vi "Set Options.vi"(8 "error in":errorcluster, 10 "WebSocket reference":refnum<class "WebSocket Client.lvclass">, 11 "Websocket Handler in":refnum<class "Websocket Handler.lvclass">) -> (0 "error out":errorcluster, 2 "reference out":refnum<class "WebSocket Client.lvclass">, 3 "Websocket Handler out":refnum<class "Websocket Handler.lvclass">)   [LabVIEW 2020, in "wamplv.lvlib" / "Websocket Handler.lvclass"]
uses:
  Websocket Handler.lvclass
  <vilib>/MediaMongrels Ltd/WebSockets/WebSockets/WebSocket Client/WebSocket Client.lvclass
  C:/Program Files (x86)/National Instruments/LabVIEW 2020/vi.lib/MediaMongrels Ltd/WebSockets/WebSockets/WebSocket/WebSocket.lvclass
  Websocket Handler.lvclass/Websocket Handler.ctl
  <vilib>/MediaMongrels Ltd/WebSockets/WebSockets/WebSocket/Headers.ctl
  <vilib>/MediaMongrels Ltd/WebSockets/WebSockets/WebSocket/WebSocket.lvclass/WebSocket.ctl
  <vilib>/MediaMongrels Ltd/WebSockets/WebSockets/WebSocket/Write Protocols.vi
  <vilib>/MediaMongrels Ltd/WebSockets/WebSockets/WebSocket/Write Send Headers.vi
  <vilib>/MediaMongrels Ltd/WebSockets/WebSockets/WebSocket/WebSocket.lvclass
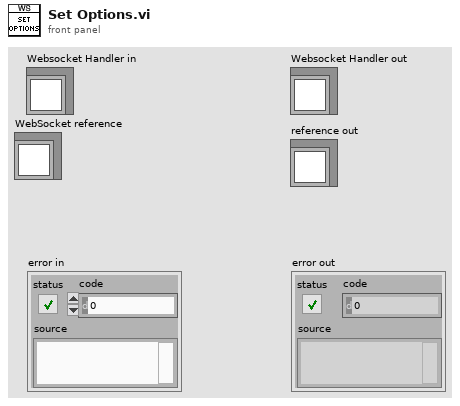
[diagram p1: front panel]
types:
  T1 = typedef "wamplv.lvlib/Websocket Handler.lvclass/Headers.ctl" = cluster{"Name":string, "Value":string}
  T2 = typedef "WebSockets.lvlib/WebSocket.lvclass/Headers.ctl" = cluster{"Name":string, "Value":string}
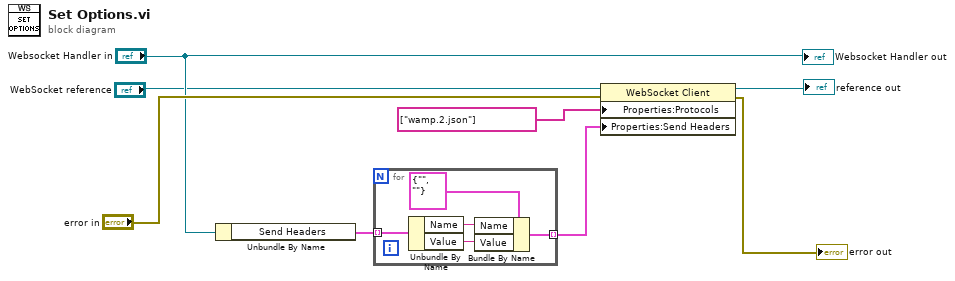
[diagram p0: block diagram]
diagram:
  n1 = Unbundle By Name("Websocket Handler in") -> ("Send Headers"=w5:T1[])
  n2 = for {
    tunnel: w5 -> [w13] mode=indexing
    tunnel: [w9] -> w2 mode=indexing
    n3 = Unbundle By Name(w13) -> ("Name"=w11:string, "Value"=w10:string)
    n4 = Bundle By Name(cluster=T2 {"Name"="", "Value"=""}, "Name"=w11, "Value"=w10) -> (w9:T2)
  }
  n5 = property class="WebSocket Client"(reference="WebSocket reference", error in="error in", "Properties:Protocols"=string[] ["wamp.2.json"] ("Protocols"), "Properties:Send Headers"=w2) -> (reference out=→"reference out":refnum<class "WebSocket Client.lvclass">, error out=→"error out":errorcluster)
  "Websocket Handler out" <- "Websocket Handler in"
